vi "Sort out Display from State.vi"(4 "func":refnum<vi>, 6 "Starting Phase":refnum<vi>, 7 "Data In":T1, 8 "error in (no error)":errorcluster, 9 "Display":refnum<vi>, 10 "Controls":refnum<vi>, 11 "Display State In":T2={"Show Axes"=FALSE, "Show Y=0"=FALSE, "Controls"={"Type"=enum."Sine", "Periods"=0.0, "Points"=0, "Offset"=0.0, "Amplitdue"=0.0, "Starting Phase"=0.0, "func"=""}, "Show Current Location"=FALSE, "Current Location"=0, "dt"=0.0, "t0"=timestamp(0 s since 1904-01-01), "Amplitude Format String"="%_3p"} caption="State" {"Controls"."Points" format="%_3p"}) -> (0 "errorout":errorcluster, 3 "Display State In 2":T2={"Show Axes"=FALSE, "Show Y=0"=FALSE, "Controls"={"Type"=enum."Sine", "Periods"=0.0, "Points"=0, "Offset"=0.0, "Amplitdue"=0.0, "Starting Phase"=0.0, "func"=""}, "Show Current Location"=FALSE, "Current Location"=0, "dt"=0.0, "t0"=timestamp(0 s since 1904-01-01), "Amplitude Format String"="%_3p"} caption="State" {"Controls"."Points" format="%_3p"})   [LabVIEW 2012, in "Waveform Control.xctl"]
uses:
  Waveform Control.xctl
  Controls/Waveform State.ctl
  FP Controls.ctl
  Function Types.ctl
  Controls/Data.ctl
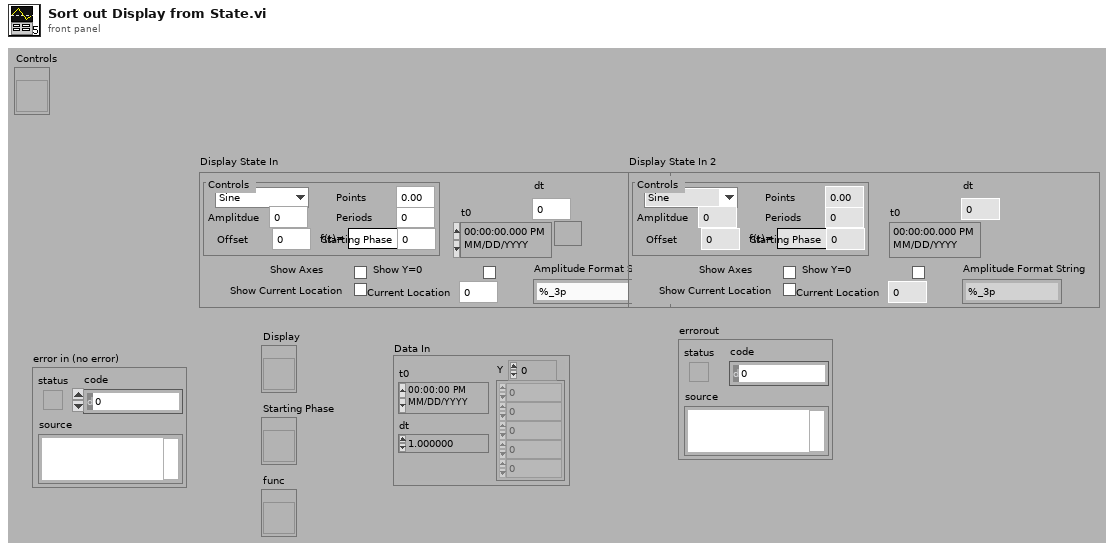
[diagram p1: front panel]
types:
  T1 = typedef "Waveform Control.xctl/Data.ctl" = waveform(dbl)
  T2 = typedef "Waveform Control.xctl/Waveform State.ctl" = cluster{"Show Axes":bool, "Show Y=0":bool, "Controls":T3, "Show Current Location":bool, "Current Location":i32, "dt":dbl, "t0":timestamp, "Amplitude Format String":string}
  T3 = typedef "Waveform Control.xctl/FP Controls.ctl" = cluster{"Type":T4, "Periods":dbl, "Points":i32, "Offset":dbl, "Amplitdue":dbl, "Starting Phase":dbl, "func":string}
  T4 = typedef "Waveform Control.xctl/Function Types.ctl" = enum16{"Level", "Sine", "Triangle", "Ramp", "Saw Tooth", "Square", "Function"}
  T5 = cluster{"Show Axes":bool, "Show Y=0":bool, "Controls":cluster{"Type":bool, "Periods":bool, "Points":bool, "Offset":bool, "Amplitdue":bool, "Starting Phase":bool, "func":bool}, "Show Current Location":bool, "Current Location":bool, "dt":bool, "t0":bool, "Amplitude Format String":bool}
  T6 = cluster{"Type":bool, "Periods":bool, "Points":bool, "Offset":bool, "Amplitdue":bool, "Starting Phase":bool, "func":bool}
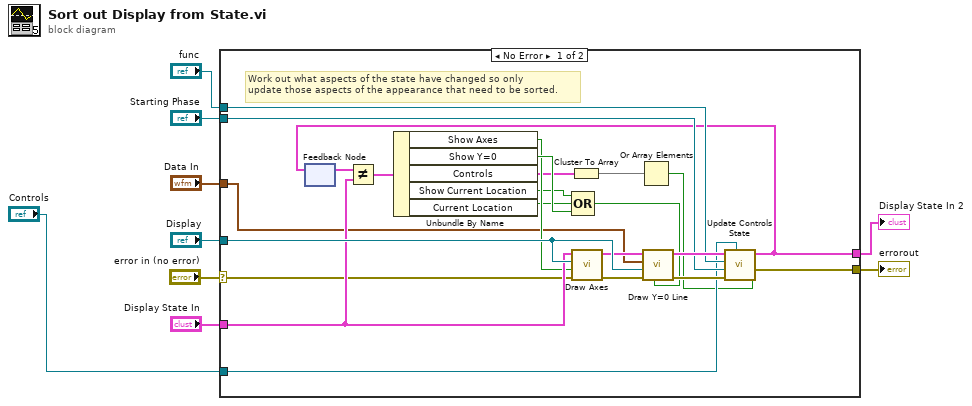
[diagram p0: block diagram]
diagram:
  n1 = case shown="No Error" "error in (no error)" {
    selector: "error in (no error)" -> [w28 w34]
    tunnel: "Display" -> [w31 _]
    tunnel: "Display State In" -> [w29 w33]
    tunnel: "Starting Phase" -> [w24 _]
    tunnel: "func" -> [w23 _]
    tunnel: "Controls" -> [w22 _]
    tunnel: [w21 w34] -> w4
    tunnel: [w11 w33] -> w3
    tunnel: "Data In" -> [w13 _]
    frame No Error {
      # "Work out what aspects of the state have changed so only\nupdate those aspects of the appearance that need to be sorted."
      n2 = feedback #1() -> (w12:T2)  [unwired: 1 out]
      n3 = Not Equal?(x=w12, y=w29) -> (x != y?=w14:T5)
      n4 = Unbundle By Name(w14) -> ("Show Axes"=w20:bool, "Show Y=0"=w32:bool, "Controls"=w17:T6, "Show Current Location"=w16:bool, "Current Location"=w15:bool)
      n5 = Cluster To Array(cluster=w17) -> (array=w18:bool[])
      n6 = Compound Arithmetic op=OR(w16, w15, w32) -> (w10:bool)
      n7 = call "Draw Axes.vi"("error in (no error)"=w28, "Show Axes"=w20, "WFGraph Refnum"=w31, "Display State In"=w29) -> ("error out"=w27:errorcluster, "Display State Out"=w30:T2)  [unwired: 6 out]
      n8 = Or Array Elements(Boolean array=w18) -> (logical OR=w19:bool)
      n9 = call "Draw Y=0 Line.vi"("Needs update"=w10, "error in (no error)"=w27, "PreviewGraph Ref"=w31, "Data In"=w13, "Display State In"=w30) -> ("error ou"=w26:errorcluster, "Display State Out"=w25:T2)  [unwired: 2 in, 3 out]
      n10 = call "Update Controls State.vi"("Controls need Update"=w19, "Controlst"=w22, "error in (no error)"=w26, "DigNum Refnum"=w24, "Str Refnum"=w23, "Display State In 2"=w25) -> ("errorout"=w21:errorcluster, "Display State In"=w11:T2)  [unwired: 4 out]
      n11 = feedback-in #1(w11) -> ()
    }
    frame Error {
    }
  }
  "errorout" <- w4
  "Display State In 2" <- w3
